vi "VISA status.vi"(8 "error in (no error)":errorcluster, 11 "AOTF in":refnum<class "Invivo_AOTF.lvclass">) -> (0 "error out":errorcluster, 3 "AOTF out":refnum<class "Invivo_AOTF.lvclass">)   [LabVIEW 2012, in "Invivo_AOTF.lvclass"]
uses:
  Invivo_AOTF.lvclass
  Invivo_AOTF.lvclass/Invivo_AOTF.ctl
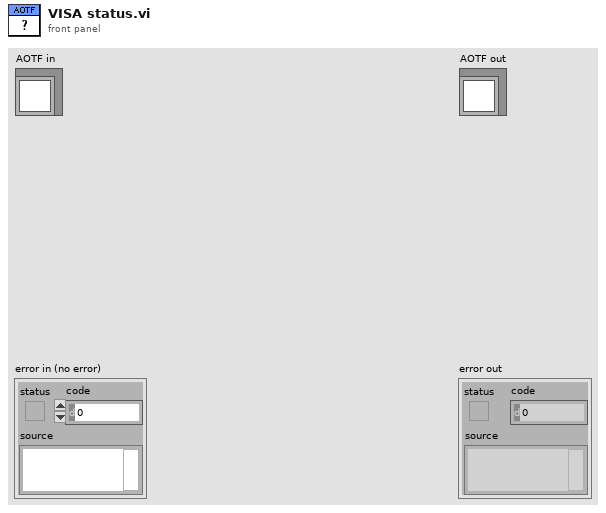
[diagram p1: front panel]
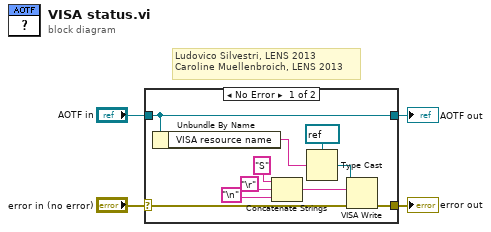
[diagram p0: block diagram]
diagram:
  # "Ludovico Silvestri, LENS 2013\nCaroline Muellenbroich, LENS 2013"
  n1 = case shown="No Error" "error in (no error)" {
    selector: "error in (no error)" -> [w7 w16]
    tunnel: [w6 w16] -> w3
    tunnel: [w5 w15] -> w1
    tunnel: "AOTF in" -> [w5 w15]
    frame No Error {
      n2 = Unbundle By Name(w5) -> ("VISA resource name"=w13:string)
      n3 = Concatenate Strings("S" ("string"), "\r", "\n") -> (w9:string)
      n4 = Type Cast(type=refnum<visa-resource-name> refnum ("VISA resource name"), x=w13) -> (*(type *) &x=w10:refnum<visa-resource-name>)
      n5 = VISA Write(VISA resource name=w10, write buffer=w9, error in (no error)=w7) -> (error out=w6:errorcluster)  [unwired: 2 out]
    }
    frame Error {
    }
  }
  "error out" <- w3
  "AOTF out" <- w1
